vi "Text_to_binary_signal_array.vi"(9 "Sampling rate (Hz)":dbl, 10 "TTL binary step duration (ms)":dbl, 11 "Text":string) -> (3 "Signal array":bool[](array[boolean]))   [LabVIEW 2016]
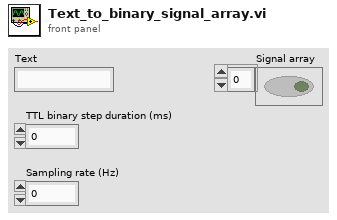
[diagram p1: front panel]
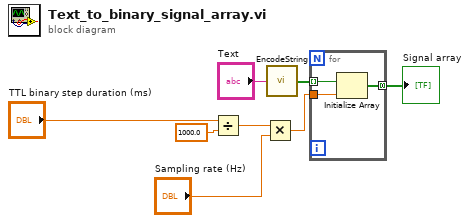
[diagram p0: block diagram]
diagram:
  n1 = Divide(x="TTL binary step duration (ms)", y=1000.0) -> (x/y=w2:dbl)
  n2 = Multiply(x=w2, y="Sampling rate (Hz)") -> (x*y=w4:dbl)
  n3 = call "EncodeString.vi"("string"="Text") -> ("Boolean array"=w3:bool[])
  n4 = for {
    tunnel: w3 -> [w11] mode=indexing
    tunnel: w4 -> [w10]
    tunnel: [w9] -> w5 mode=concatenating
    n5 = Initialize Array(w11, w10) -> (w9:bool[])
  }
  "Signal array" <- w5
